vi "Get Result.vi"(8 "error in (no error)":errorcluster, 11 "NI-Scope Lock-in Driver in":refnum<class "NI-Scope Lock-in Driver.lvclass">) -> (0 "error out":errorcluster, 2 "Result":refnum<class "Acquired Result.lvclass">, 3 "NI-Scope Lock-in Driver out":refnum<class "NI-Scope Lock-in Driver.lvclass">)   [LabVIEW 2016, in "NI-Scope Lock-in Driver.lvclass"]
uses:
  NI-Scope Lock-in Driver.lvclass
  C:/github/NHMFL_Core/Libraries/Instruments/Pulse Driver/Pulse Driver.lvclass
  Instruments/Results/Acquired Result/Acquired Result.lvclass
  NI-Scope Lock-in Driver.lvclass/NI-Scope Lock-in Driver.ctl
  Instruments/Pulse Driver/Pulse Driver.lvclass/Pulse Driver.ctl
  Read Sine.vi
  Read Cosine.vi
  Instruments/Pulse Driver/Write Samples per read.vi
panel:
  out "Waveform Graph":i16[][](graph)
  out "Current read position":i32
  out "Availiable Samples":u32
  out "Sine waves read":dbl format="%.6g"
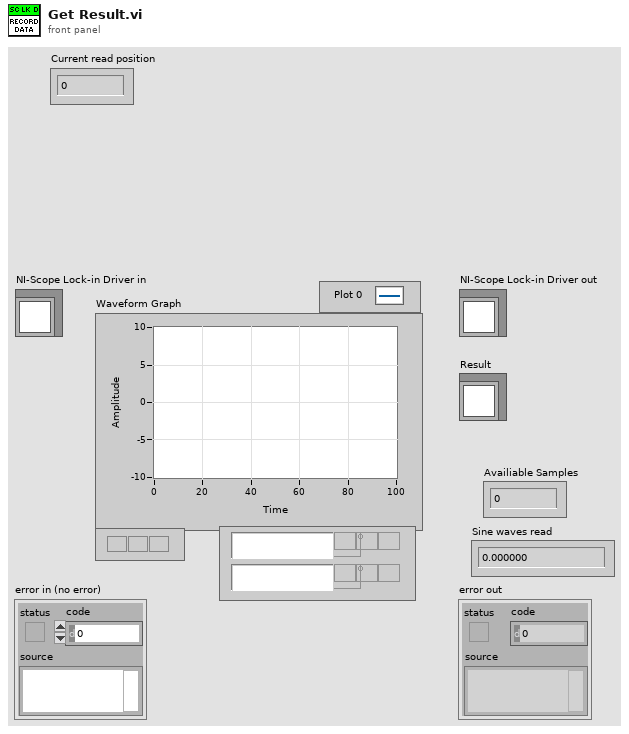
[diagram p1: front panel]
types:
  T1 = typedef "NI-Scope Lock-in Configuration.ctl" = cluster{"Points per sine wave":i32, "Rate":dbl, "Re-name channels":string[], "Active channels":string, "Ranges":dbl[], "Sync on trigger":bool}
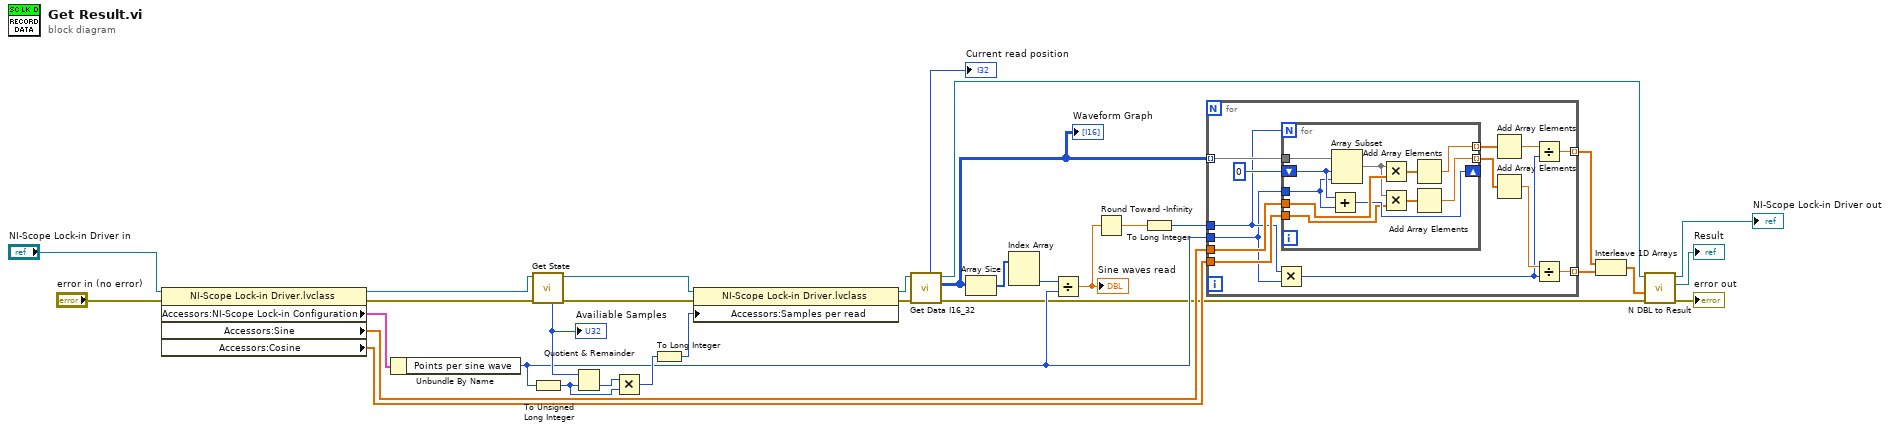
[diagram p0: block diagram]
diagram:
  n1 = property class="NI-Scope Lock-in Driver.lvclass"(reference="NI-Scope Lock-in Driver in", error in="error in (no error)") -> (reference out=w18:refnum<class "NI-Scope Lock-in Driver.lvclass">, error out=w3:errorcluster, "Accessors:NI-Scope Lock-in Configuration"=w17:T1, "Accessors:Sine"=w13:dbl[], "Accessors:Cosine"=w9:dbl[])
  n2 = Unbundle By Name(w17) -> ("Points per sine wave"=w14:i32)
  n3 = call-dynamic "Get State.vi"("error in (no error)"=w3, "NI-Scope Lock-in Driver in"=w18) -> ("error out"=w27:errorcluster, "NI-Scope Lock-in Driver out"=w29:refnum<class "NI-Scope Lock-in Driver.lvclass">, "Availiable Samples"=w30:u32)  [unwired: 4 in, 3 out]
  "Availiable Samples" <- w30
  n4 = To Unsigned Long Integer(number=w14) -> (unsigned 32bit integer=w24:u32)
  n5 = Quotient & Remainder(x=w30, y=w24) -> (floor(x/y)=w25:u32)  [unwired: 1 out]
  n6 = Multiply(x=w25, y=w24) -> (x*y=w23:u32)
  n7 = To Long Integer(number=w23) -> (32bit integer=w22:i32)
  n8 = property class="NI-Scope Lock-in Driver.lvclass"(reference=w29, error in=w27, "Accessors:Samples per read"=w22) -> (reference out=w28:refnum<class "NI-Scope Lock-in Driver.lvclass">, error out=w26:errorcluster)
  n9 = call-dynamic "Get Data I16_32.vi"("error in (no error)"=w26, "Ni-Scope Digitizer in"=w28) -> ("error out"=w7:errorcluster, "I16 data out"=w1:i16[][], "Ni-Scope Digitizer out"=w12:refnum<class "NI-Scope Lock-in Driver.lvclass">, "Current read position"=→"Current read position":i32)  [unwired: 4 in, 2 out]
  "Waveform Graph" <- w1
  n10 = Array Size(array=w1) -> (size(s)=w21:i32[])
  n11 = Index Array(array=w21) -> (element #2=w20:i32)  [unwired: 2 in, 1 out]
  n12 = Divide(x=w20, y=w14) -> (x/y=w16:dbl)
  "Sine waves read" <- w16
  n13 = Round Toward -Infinity(1:w16) -> (0:w15:dbl)
  n14 = To Long Integer(number=w15) -> (32bit integer=w2:i32)
  n15 = for {
    tunnel: w1 -> [w45] mode=indexing
    tunnel: w14 -> [w38]
    tunnel: w13 -> [w43]
    tunnel: [w37] -> w11 mode=indexing
    tunnel: w9 -> [w40]
    tunnel: [w33] -> w8 mode=indexing
    tunnel: w2 -> [w39]
    n16 = Multiply(x=w39, y=w38) -> (x*y=w34:i32)
    n17 = for {
      N: w39 -> [_]
      tunnel: w45 -> [w56]
      shift-right: [w51] -> _
      shift-left: 0 -> [w53]
      tunnel: w38 -> [w52]
      tunnel: w43 -> [w55]
      tunnel: [w50] -> w42 mode=indexing
      tunnel: [w49] -> w41 mode=indexing
      tunnel: w40 -> [w46]
      n18 = Add(x=w53, y=w52) -> (x+y=w51:i32)
      n19 = Array Subset(array=w56, index=w53, length=w52) -> (w47:i16[])
      n20 = Multiply(x=w47, y=w55) -> (x*y=w54:dbl[])
      n21 = Multiply(x=w47, y=w46) -> (x*y=w48:dbl[])
      n22 = Add Array Elements(numeric array=w54) -> (sum=w50:dbl)
      n23 = Add Array Elements(numeric array=w48) -> (sum=w49:dbl)
    }
    n24 = Add Array Elements(numeric array=w42) -> (sum=w36:dbl)
    n25 = Add Array Elements(numeric array=w41) -> (sum=w35:dbl)
    n26 = Divide(x=w36, y=w34) -> (x/y=w37:dbl)
    n27 = Divide(x=w35, y=w34) -> (x/y=w33:dbl)
  }
  n28 = Interleave 1D Arrays(w11, w8) -> (w10:dbl[])
  n29 = call-dynamic "N DBL to Result.vi"("error in (no error)"=w7, "Data"=w10, "Instrument Driver in"=w12) -> ("error out"=→"error out":errorcluster, "Result out"=→"Result":refnum<class "Acquired Result.lvclass">, "Instrument Driver out"=→"NI-Scope Lock-in Driver out":refnum<class "NI-Scope Lock-in Driver.lvclass">)  [unwired: 6 in]
